vi "8CHDAQ - Create Channels.vi"(10 "Channel Data":T1) -> (0 "error out":errorcluster, 3 "task out":refnum<k21>)   [LabVIEW 2015]
uses:
  <vilib>/DAQmx/create/channels.llb/DAQmx Create Channel (AI-Voltage-Basic).vi
  <vilib>/DAQmx/create/channels.llb/DAQmx Create Channel (AI-Acceleration-Accelerometer).vi
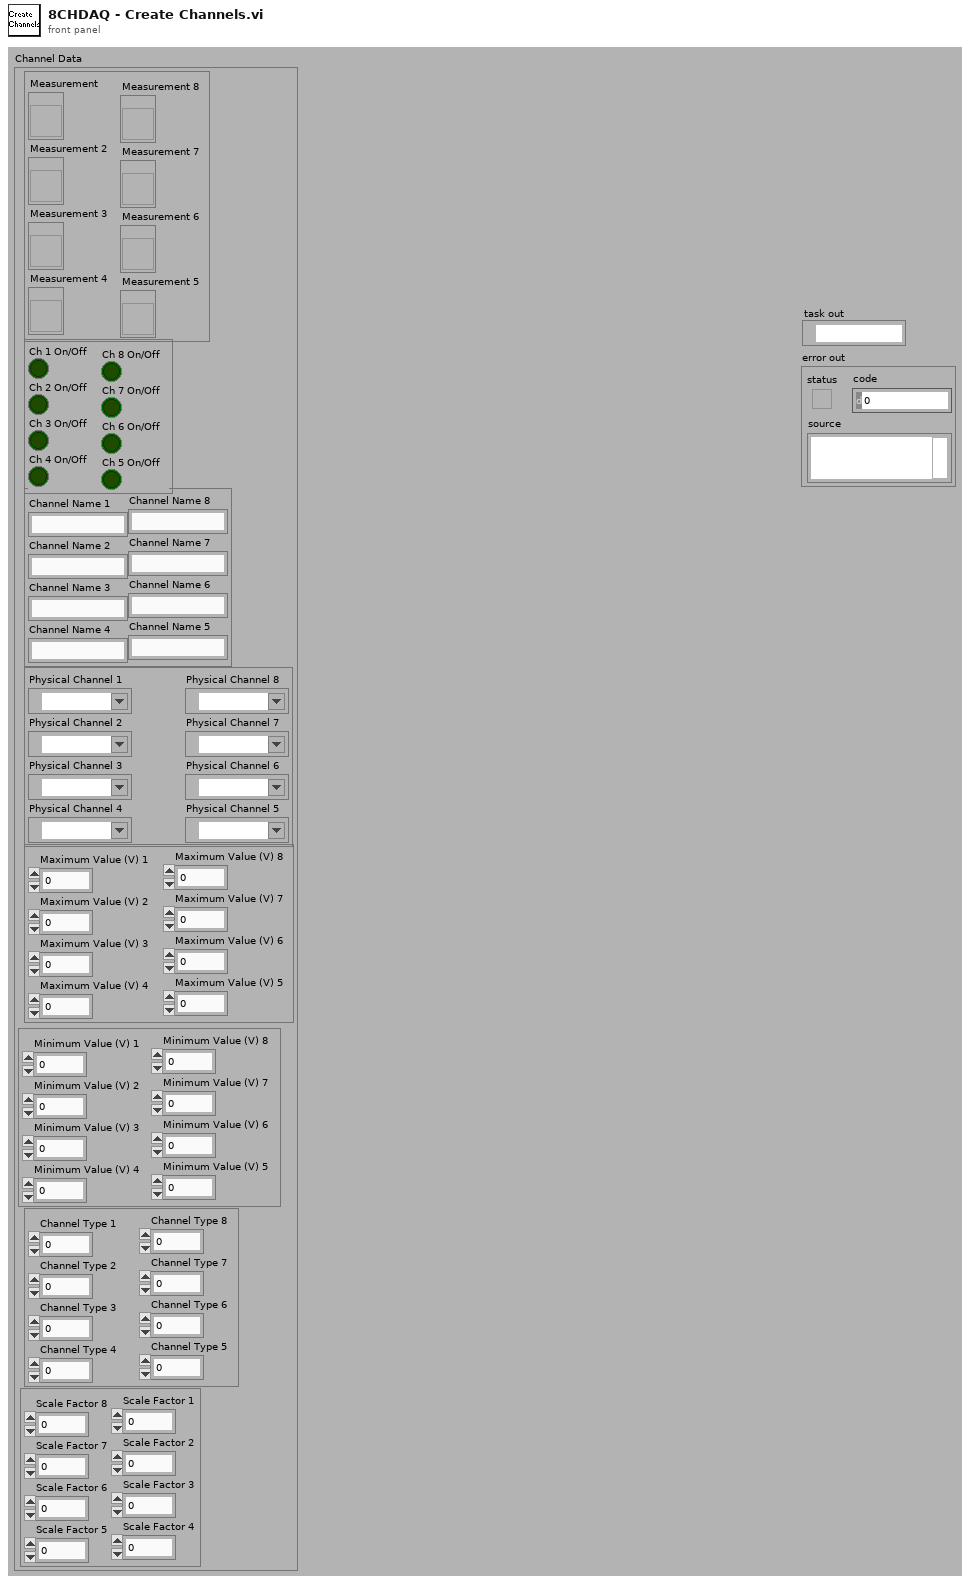
[diagram p1: front panel]
types:
  T1 = cluster{cluster{"Measurement":refnum<vi>, "Measurement 2":refnum<vi>, "Measurement 3":refnum<vi>, "Measurement 4":refnum<vi>, "Measurement 5":refnum<vi>, "Measurement 6":refnum<vi>, "Measurement 7":refnum<vi>, "Measurement 8":refnum<vi>}, cluster{"Ch 1 On/Off":bool, "Ch 2 On/Off":bool, "Ch 3 On/Off":bool, "Ch 4 On/Off":bool, "Ch 5 On/Off":bool, "Ch 6 On/Off":bool, "Ch 7 On/Off":bool, "Ch 8 On/Off":bool}, cluster{"Channel Name 1":string, "Channel Name 2":string, "Channel Name 3":string, "Channel Name 4":string, "Channel Name 5":string, "Channel Name 6":string, "Channel Name 7":string, "Channel Name 8":string}, cluster{"Physical Channel 1":tag, "Physical Channel 2":tag, "Physical Channel 3":tag, "Physical Channel 4":tag, "Physical Channel 5":tag, "Physical Channel 6":tag, "Physical Channel 7":tag, "Physical Channel 8":tag}, cluster{"Maximum Value (V) 1":dbl, "Maximum Value (V) 2":dbl, "Maximum Value (V) 3":dbl, "Maximum Value (V) 4":dbl, "Maximum Value (V) 5":dbl, "Maximum Value (V) 6":dbl, "Maximum Value (V) 7":dbl, "Maximum Value (V) 8":dbl}, cluster{"Minimum Value (V) 1":dbl, "Minimum Value (V) 2":dbl, "Minimum Value (V) 3":dbl, "Minimum Value (V) 4":dbl, "Minimum Value (V) 5":dbl, "Minimum Value (V) 6":dbl, "Minimum Value (V) 7":dbl, "Minimum Value (V) 8":dbl}, cluster{"Channel Type 1":u16, "Channel Type 2":u16, "Channel Type 3":u16, "Channel Type 4":u16, "Channel Type 5":u16, "Channel Type 6":u16, "Channel Type 7":u16, "Channel Type 8":u16}, cluster{"Scale Factor 8":dbl[unit], "Scale Factor 7":dbl[unit], "Scale Factor 6":dbl[unit], "Scale Factor 5":dbl[unit], "Scale Factor 4":dbl[unit], "Scale Factor 3":dbl[unit], "Scale Factor 2":dbl[unit], "Scale Factor 1":dbl[unit]}}
  T2 = cluster{"Ch 1 On/Off":bool, "Ch 2 On/Off":bool, "Ch 3 On/Off":bool, "Ch 4 On/Off":bool, "Ch 5 On/Off":bool, "Ch 6 On/Off":bool, "Ch 7 On/Off":bool, "Ch 8 On/Off":bool}
  T3 = cluster{"Channel Name 1":string, "Channel Name 2":string, "Channel Name 3":string, "Channel Name 4":string, "Channel Name 5":string, "Channel Name 6":string, "Channel Name 7":string, "Channel Name 8":string}
  T4 = cluster{"Physical Channel 1":tag, "Physical Channel 2":tag, "Physical Channel 3":tag, "Physical Channel 4":tag, "Physical Channel 5":tag, "Physical Channel 6":tag, "Physical Channel 7":tag, "Physical Channel 8":tag}
  T5 = cluster{"Maximum Value (V) 1":dbl, "Maximum Value (V) 2":dbl, "Maximum Value (V) 3":dbl, "Maximum Value (V) 4":dbl, "Maximum Value (V) 5":dbl, "Maximum Value (V) 6":dbl, "Maximum Value (V) 7":dbl, "Maximum Value (V) 8":dbl}
  T6 = cluster{"Minimum Value (V) 1":dbl, "Minimum Value (V) 2":dbl, "Minimum Value (V) 3":dbl, "Minimum Value (V) 4":dbl, "Minimum Value (V) 5":dbl, "Minimum Value (V) 6":dbl, "Minimum Value (V) 7":dbl, "Minimum Value (V) 8":dbl}
  T7 = cluster{"Channel Type 1":u16, "Channel Type 2":u16, "Channel Type 3":u16, "Channel Type 4":u16, "Channel Type 5":u16, "Channel Type 6":u16, "Channel Type 7":u16, "Channel Type 8":u16}
  T8 = cluster{"Scale Factor 8":dbl[unit], "Scale Factor 7":dbl[unit], "Scale Factor 6":dbl[unit], "Scale Factor 5":dbl[unit], "Scale Factor 4":dbl[unit], "Scale Factor 3":dbl[unit], "Scale Factor 2":dbl[unit], "Scale Factor 1":dbl[unit]}
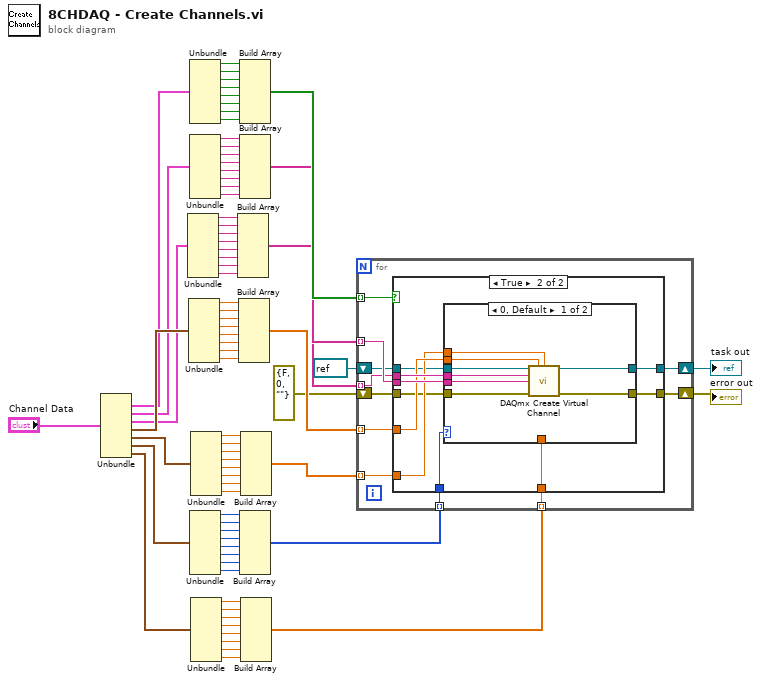
[diagram p0: block diagram]
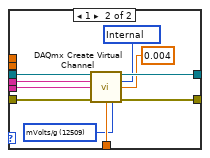
[diagram p3: hidden frame]
diagram:
  n1 = Unbundle("Channel Data") -> (w30:T2, w31:T3, w32:T4, w33:T5, w34:T6, w35:T7, w36:T8)  [unwired: 1 out]
  n2 = Unbundle(w32) -> ("Physical Channel 1"=w66:tag, "Physical Channel 2"=w65:tag, "Physical Channel 3"=w64:tag, "Physical Channel 4"=w63:tag, "Physical Channel 5"=w4:tag, "Physical Channel 6"=w3:tag, "Physical Channel 7"=w2:tag, "Physical Channel 8"=w1:tag)
  n3 = Unbundle(w33) -> ("Maximum Value (V) 1"=w59:dbl, "Maximum Value (V) 2"=w60:dbl, "Maximum Value (V) 3"=w61:dbl, "Maximum Value (V) 4"=w62:dbl, "Maximum Value (V) 5"=w15:dbl, "Maximum Value (V) 6"=w14:dbl, "Maximum Value (V) 7"=w13:dbl, "Maximum Value (V) 8"=w16:dbl)
  n4 = Unbundle(w30) -> ("Ch 1 On/Off"=w75:bool, "Ch 2 On/Off"=w74:bool, "Ch 3 On/Off"=w73:bool, "Ch 4 On/Off"=w72:bool, "Ch 5 On/Off"=w24:bool, "Ch 6 On/Off"=w23:bool, "Ch 7 On/Off"=w22:bool, "Ch 8 On/Off"=w21:bool)
  n5 = Unbundle(w31) -> ("Channel Name 1"=w67:string, "Channel Name 2"=w68:string, "Channel Name 3"=w69:string, "Channel Name 4"=w70:string, "Channel Name 5"=w28:string, "Channel Name 6"=w27:string, "Channel Name 7"=w26:string, "Channel Name 8"=w25:string)
  n6 = Unbundle(w35) -> ("Channel Type 1"=w43:u16, "Channel Type 2"=w44:u16, "Channel Type 3"=w45:u16, "Channel Type 4"=w46:u16, "Channel Type 5"=w12:u16, "Channel Type 6"=w11:u16, "Channel Type 7"=w9:u16, "Channel Type 8"=w10:u16)
  n7 = Unbundle(w34) -> ("Minimum Value (V) 1"=w58:dbl, "Minimum Value (V) 2"=w57:dbl, "Minimum Value (V) 3"=w56:dbl, "Minimum Value (V) 4"=w55:dbl, "Minimum Value (V) 5"=w20:dbl, "Minimum Value (V) 6"=w19:dbl, "Minimum Value (V) 7"=w18:dbl, "Minimum Value (V) 8"=w17:dbl)
  n8 = Unbundle(w36) -> ("Scale Factor 8"=w42:dbl[unit], "Scale Factor 7"=w41:dbl[unit], "Scale Factor 6"=w40:dbl[unit], "Scale Factor 5"=w39:dbl[unit], "Scale Factor 4"=w8:dbl[unit], "Scale Factor 3"=w7:dbl[unit], "Scale Factor 2"=w6:dbl[unit], "Scale Factor 1"=w5:dbl[unit])
  n9 = Build Array(w66, w65, w64, w63, w4, w3, w2, w1) -> (w53:tag[])
  n10 = Build Array(w59, w60, w61, w62, w15, w14, w13, w16) -> (w52:dbl[])
  n11 = Build Array(w75, w74, w73, w72, w24, w23, w22, w21) -> (w71:bool[])
  n12 = Build Array(w67, w68, w69, w70, w28, w27, w26, w25) -> (w54:string[])
  n13 = Build Array(w43, w44, w45, w46, w12, w11, w9, w10) -> (w38:u16[])
  n14 = Build Array(w58, w57, w56, w55, w20, w19, w18, w17) -> (w51:dbl[])
  n15 = Build Array(w42, w41, w40, w39, w8, w7, w6, w5) -> (w37:dbl[])
  n16 = for {
    tunnel: w71 -> [w86] mode=indexing
    tunnel: w54 -> [w85] mode=indexing
    tunnel: w53 -> [w84] mode=indexing
    tunnel: w52 -> [w83] mode=indexing
    tunnel: w51 -> [w82] mode=indexing
    shift-right: [w81] -> w48
    shift-left: refnum<k21> refnum ("task out") -> [w79]
    shift-right: [w80] -> w47
    shift-left: errorcluster {"status"=FALSE, "code"=0, "source"=""} ("error out") -> [w78]
    tunnel: w38 -> [w77] mode=indexing
    tunnel: w37 -> [w76] mode=indexing
    n17 = case shown="True" w86 {
      tunnel: w85 -> [_ w98]
      tunnel: w84 -> [_ w97]
      tunnel: w83 -> [_ w96]
      tunnel: w82 -> [_ w95]
      tunnel: [w88 w94] -> w81
      tunnel: [w87 w93] -> w80
      tunnel: w79 -> [w88 w92]
      tunnel: w78 -> [w87 w91]
      tunnel: w77 -> [_ w90]
      tunnel: w76 -> [_ w89]
      frame False {
      }
      frame True {
        n18 = case shown="0, Default" w90 {
          tunnel: w98 -> [w106 w110]
          tunnel: w97 -> [w105 w111]
          tunnel: w96 -> [w104 _]
          tunnel: w95 -> [w103 _]
          tunnel: [w102 w116] -> w94
          tunnel: [w101 w115] -> w93
          tunnel: w92 -> [w100 w113]
          tunnel: w91 -> [w99 w112]
          tunnel: w89 -> [_ w114]
          frame 0, Default {
            n19 = call-poly <vilib>:"DAQmx Create Virtual Channel.vi"("task in"=w100, "maximum value"=w104, "minimum value"=w103, "physical channels"=w105, "name to assign"=w106, "error in"=w99) -> ("task out"=w102:refnum<k21>, "error out"=w101:errorcluster)  [unwired: 8 in]
          }
          frame 1 {
            w107 = 12509 items=["mVolts/g"=12509, "Volts/g"=12510] ("sensitivity units")
            w109 = 10200 items=["Internal"=10200, "External"=10167, "None"=10230] ("current excitation source")
            n20 = call-poly <vilib>:"DAQmx Create Virtual Channel.vi"("task in"=w113, "physical channels"=w111, "current excitation source"=w109, "name to assign"=w110, "current excitation value"=0.004, "error in"=w112, "sensitivity"=w114, "sensitivity units"=w107) -> ("task out"=w116:refnum<k21>, "error out"=w115:errorcluster)  [unwired: 6 in]
          }
        }
      }
    }
  }
  "task out" <- w48
  "error out" <- w47
